vi "testing_test1.vi"() -> ()   [LabVIEW 2015]
uses:
  <vilib>/LabVIEW Interface for Arduino/LabVIEW Interface for Arduino.lvlib
panel:
  out "Tab Control":T1(tab)
  out "?":string
  in  "Exit the program":bool
  in  "Start Test":bool
  in  "Next Button 2":bool
  out "String 2":string
  in  "Next Button 3":bool
  out "String 3":string
  in  "stop 2":bool
  in  "Next Button 4":bool
  out "String 4":string
  in  "stop K1":bool
  out "Error":string
  out "Last  Message":string
  in  "Complete K1":bool
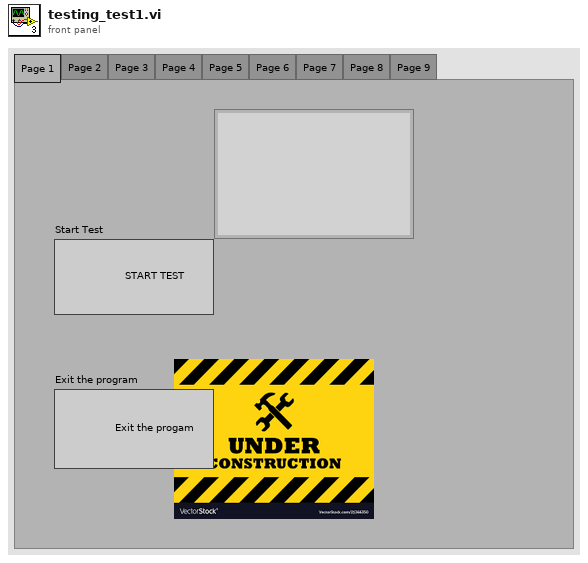
[diagram p1: front panel]
types:
  T1 = enum32{"Page 1", "Page 2", "Page 3", "Page 4", "Page 5", "Page 6", "Page 7", "Page 8", "Page 9"}
  T2 = typedef "LabVIEW Interface for Arduino.lvlib/Arduino Resource.ctl" = cluster{"VISA resource":refnum<visa-resource-name>, "Board Type":T3, "Connection Type":enum8{"USB / Serial"}, "Bytes Per Packet (15)":u8}
  T3 = typedef "LabVIEW Interface for Arduino.lvlib/Board Type.ctl" = enum16{"Uno", "Dimuelanove w/Atmega 328", "Mega 2560"}
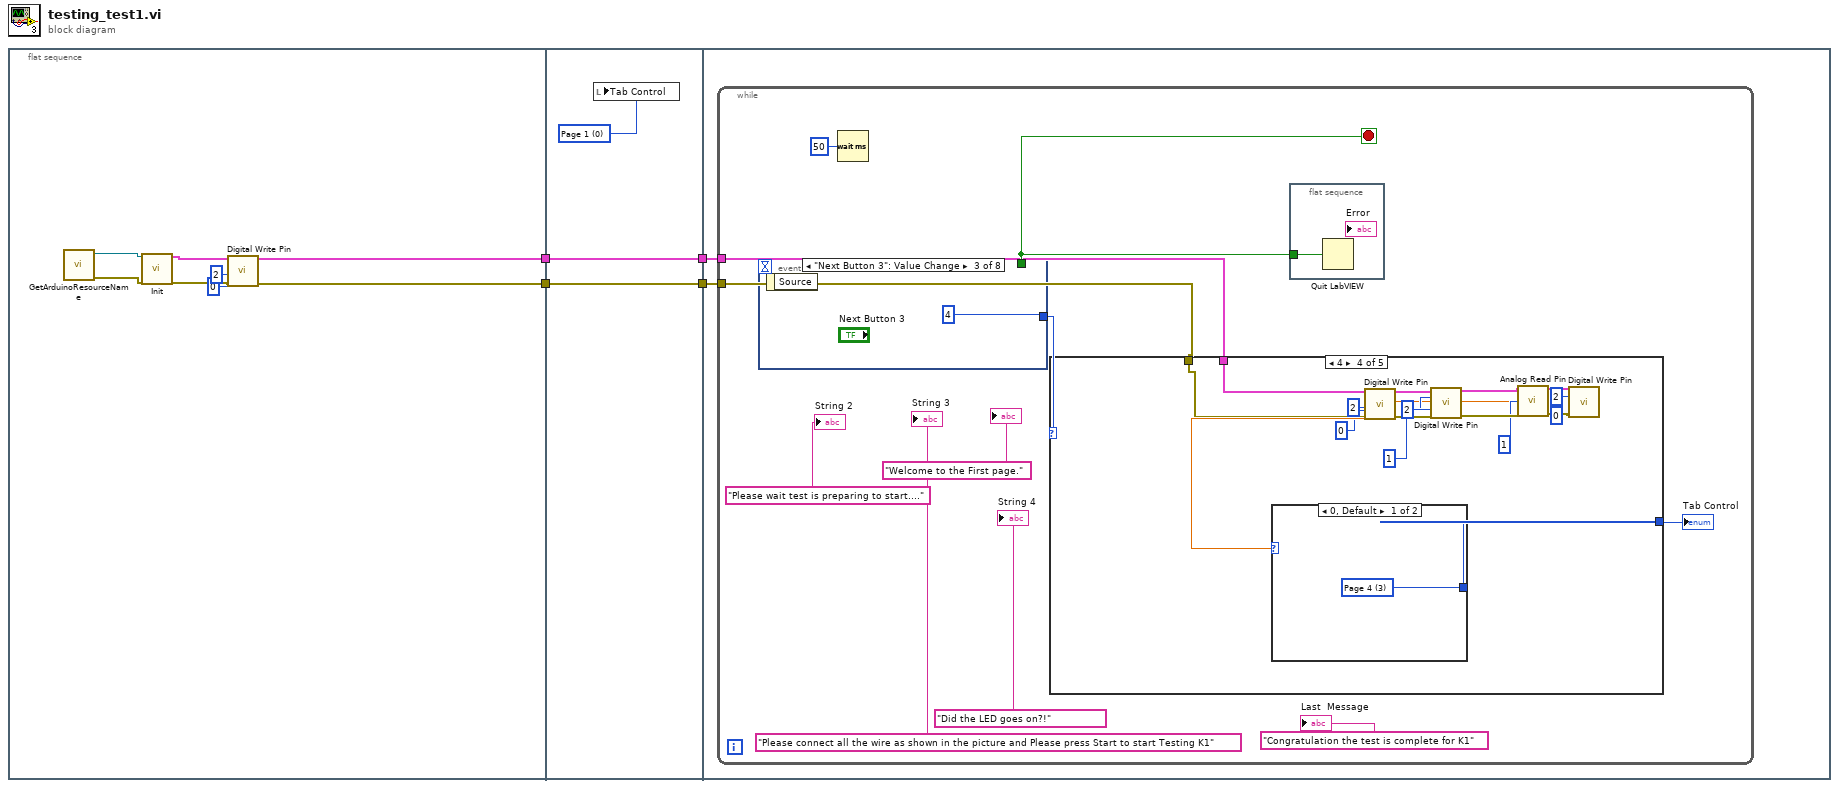
[diagram p0: block diagram]
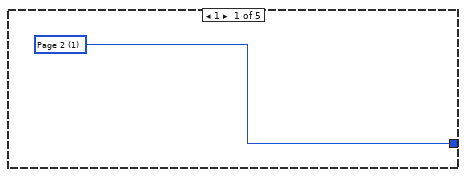
[diagram p2: hidden frame]
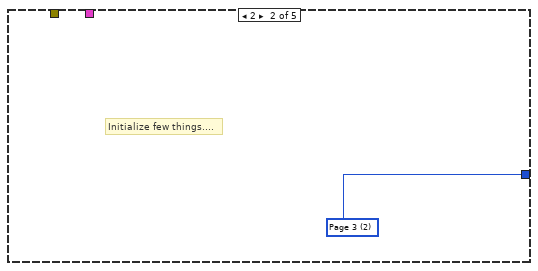
[diagram p3: hidden frame]
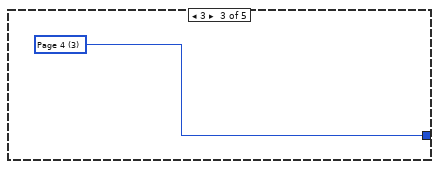
[diagram p4: hidden frame]
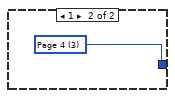
[diagram p5: hidden frame]
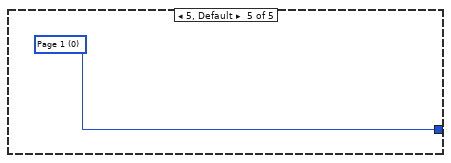
[diagram p6: hidden frame]
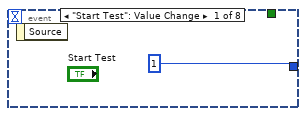
[diagram p7: hidden frame]
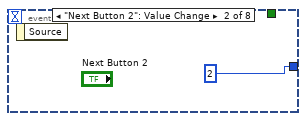
[diagram p8: hidden frame]
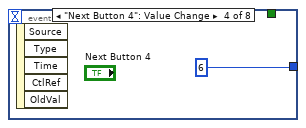
[diagram p9: hidden frame]
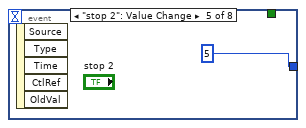
[diagram p10: hidden frame]
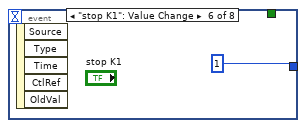
[diagram p11: hidden frame]
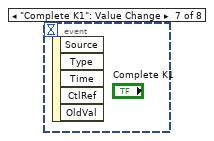
[diagram p12: hidden frame]
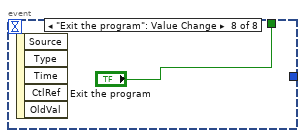
[diagram p13: hidden frame]
diagram:
  n1 = flat-sequence {
    tunnel: [w6] -> w3
    tunnel: [w5] -> w1
    tunnel: [w14] -> w4
    tunnel: w3 -> [w14]
    tunnel: [w13] -> w2
    tunnel: w1 -> [w13]
    tunnel: w4 -> [w17]
    tunnel: w2 -> [w16]
    frame #0 {
      n2 = call "GetArduinoResourceName.vi"() -> ("error out"=w7:errorcluster, "VISA resource name"=w8:refnum<visa-resource-name>)  [unwired: 10 in]
      n3 = call <vilib>:"Init.vi"("VISA resource"=w8, "error in"=w7) -> ("Arduino Resource"=w12:T2, "error out"=w11:errorcluster)  [unwired: 16 in]
      n4 = call <vilib>:"Digital Write Pin.vi"("Arduino Resource"=w12, "Digital I/O Pin (0)"=u8 2 ("Digital I/O Pin"), "Value (0)"=u8 0, "error in"=w11) -> ("Arduino Resource"=w6:T2, "error out"=w5:errorcluster)  [unwired: 10 in]
    }
    frame #1 {
      w15 = u16 0 items=["Page 1"]
      n5 = local write "Tab Control"(w15) -> ()
    }
    frame #2 {
      n6 = while {
        tunnel: w17 -> [w18]
        tunnel: w16 -> [w19]
        stop <- w23 stop-if-true
        n7 = event shown="[2] \"Next Button 3\": Value Change" {
          selector: _ -> [_ _ _ _ _ _ _ _]
          dyn-events: _ -> [_ _ _ _ _ _ _ _]
          timeout: _ -> [_ _ _ _ _ _ _ _]
          tunnel: [1 2 4 6 5 1 _ _] -> w27
          tunnel: [_ _ _ _ _ _ _ "Exit the program"] -> w23
          event "Start Test": Value Change {
            n8 = event-data() -> ()  [unwired: 1 in, 1 out]
          }
          event "Next Button 2": Value Change {
            n9 = event-data() -> ()  [unwired: 1 in, 1 out]
          }
          event "Next Button 3": Value Change {
            n10 = event-data() -> ()  [unwired: 1 in, 1 out]
          }
          event "Next Button 4": Value Change {
            n11 = event-data() -> ()  [unwired: 1 in, 5 out]
          }
          event "stop 2": Value Change {
            n12 = event-data() -> ()  [unwired: 1 in, 5 out]
          }
          event "stop K1": Value Change {
            n13 = event-data() -> ()  [unwired: 1 in, 5 out]
          }
          event "Complete K1": Value Change {
            n14 = event-data() -> ()  [unwired: 1 in, 5 out]
          }
          event "Exit the program": Value Change {
            n15 = event-data() -> ()  [unwired: 1 in, 5 out]
          }
        }
        n16 = Wait (ms)(milliseconds to wait=u32 50) -> ()  [unwired: 1 out]
        n17 = case shown="4" w27 {
          tunnel: [w29 w30 w31 w39 w51] -> w21
          tunnel: w19 -> [_ _ _ w33 _]
          tunnel: w18 -> [_ _ _ w34 _]
          frame 1 {
            w29 = u16 1 items=["Page 1", "Page 2", "Page 3"]
          }
          frame 2 {
            w30 = u16 2 items=["Page 1", "Page 2", "Page 3", "Page 4"]
            # "Initialize few things...."
          }
          frame 3 {
            w31 = u16 3 items=["Page 1", "Page 2", "Page 3", "Page 4", "Page 5"]
          }
          frame 4 {
            n18 = call <vilib>:"Digital Write Pin.vi"("Arduino Resource"=w34, "Digital I/O Pin (0)"=u8 2 ("Digital I/O Pin"), "Value (0)"=u8 0, "error in"=w33) -> ("Arduino Resource"=w48:T2, "error out"=w47:errorcluster)  [unwired: 10 in]
            n19 = call <vilib>:"Digital Write Pin.vi"("Arduino Resource"=w48, "Digital I/O Pin (0)"=u8 2, "Value (0)"=u8 1, "error in"=w47) -> ("Arduino Resource"=w43:T2, "error out"=w42:errorcluster)  [unwired: 10 in]
            n20 = call <vilib>:"Analog Read Pin.vi"("Arduino Resource"=w43, "Analog Input Pin (0)"=u8 1, "error in"=w42) -> ("Arduino Resource"=w38:T2, "Voltage"=w40:dbl, "error out"=w37:errorcluster)  [unwired: 10 in]
            n21 = case shown="0, Default" w40 {
              tunnel: [w49 w50] -> w39
              frame 0, Default {
                w49 = u16 3 items=["Page 1", "Page 2", "Page 3", "Page 4", "Page 5", "Page 6"]
              }
              frame 1 {
                w50 = u16 3 items=["Page 1", "Page 2", "Page 3", "Page 4", "Page 5", "Page 6"]
              }
            }
            n22 = call <vilib>:"Digital Write Pin.vi"("Arduino Resource"=w38, "Digital I/O Pin (0)"=u8 2, "Value (0)"=u8 0, "error in"=w37) -> ()  [unwired: 10 in, 2 out]
          }
          frame 5, Default {
            w51 = u16 0 items=["Page 1"]
          }
        }
        "Tab Control" <- w21
        n23 = flat-sequence {
          tunnel: w23 -> [w59]
          frame #0 {
            n24 = Quit LabVIEW(quit? (T)=w59) -> ()
          }
        }
        "?" <- "Welcome to the First page."
        "String 2" <- "Please wait test is preparing to start...."
        "String 3" <- "Please connect all the wire as shown in the picture and Please press Start to start Testing K1"
        "String 4" <- "Did the LED goes on?!"
        "Last  Message" <- "Congratulation the test is complete for K1" ("Last  Message")
      }
    }
  }
